vi "CSV reader.vi"(9 "x":dbl, 10 "Array":string[](array[string]), 11 "Number CSV":dbl) -> (1 "Auton Array":dbl[][](array[numeric]), 2 "File Selected":string)   [LabVIEW 2014]
uses:
  <vilib>/Utility/file.llb/Read From Spreadsheet File (DBL).vi
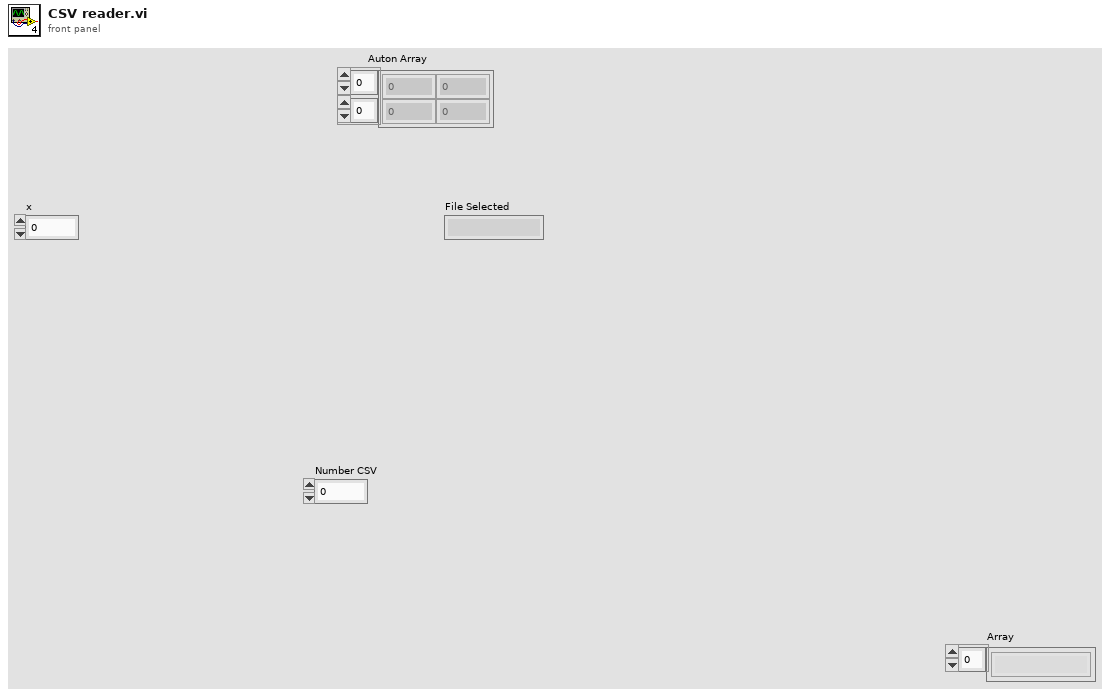
[diagram p1: front panel]
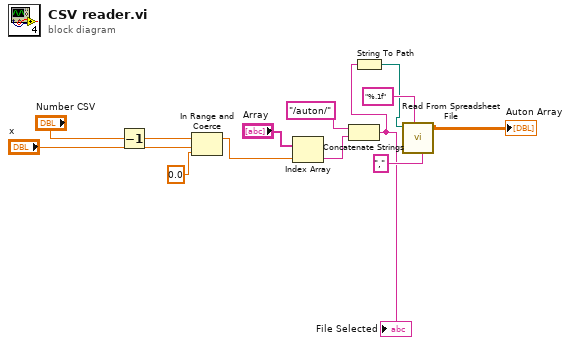
[diagram p0: block diagram]
diagram:
  n1 = Decrement(x="Number CSV") -> (x-1=w10:dbl)
  n2 = In Range and Coerce(upper limit=w10, x="x", lower limit=0.0) -> (coerced(x)=w7:dbl)  [unwired: 1 out]
  n3 = Index Array(array="Array", index=w7) -> (element=w5:string)
  n4 = Concatenate Strings("/auton/" ("string"), w5) -> (w3:string)
  "File Selected" <- w3
  n5 = String To Path(string=w3) -> (path=w2:path)
  n6 = call-poly <vilib>:"Read From Spreadsheet File.vi"("delimiter (\\t)"="," ("delimiter (\\t)"), "format (%.3f)"="%.1f", "file path (dialog if empty)"=w2) -> ("all rows"=→"Auton Array":dbl[][])  [unwired: 4 in, 4 out]
